vi "read-write user data.vi"(7 "Function":enum16{"Read", "Write"}(ring), 8 "error in (no error)":errorcluster, 10 "user data in":T1={"sectors"=[], "key names"=[], "values"=[]}, 11 "file name":string) -> (0 "error out":errorcluster, 2 "user data out":T1)   [LabVIEW 2015]
doc: "This VI saves (Write) and retrieves (Read) data from a configuration .ini file, regardless of the number of sectors and the keys in each sector."
uses:
  <vilib>/Utility/config.llb/NI_LVConfig.lvlib
  <vilib>/Utility/config.llb/Read Key (String).vi
  <vilib>/Utility/config.llb/Write Key (String).vi
  controls/user data.ctl
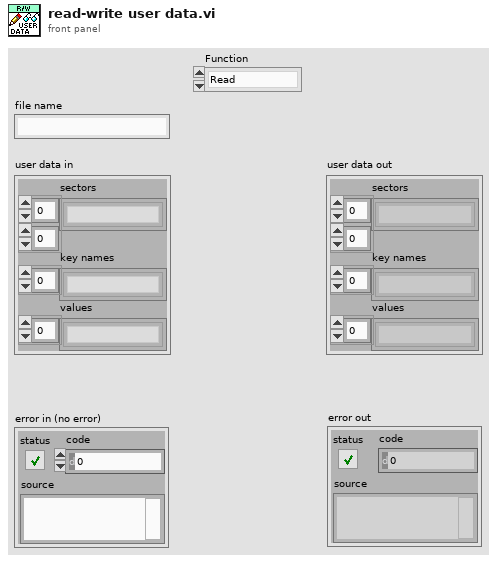
[diagram p1: front panel]
types:
  T1 = typedef "user data.ctl" = cluster{"sectors":string[][], "key names":string[], "values":string[]}
  T2 = typedef "NI_LVConfig.lvlib/Config Data RefNum.ctl" = refnum<k1>
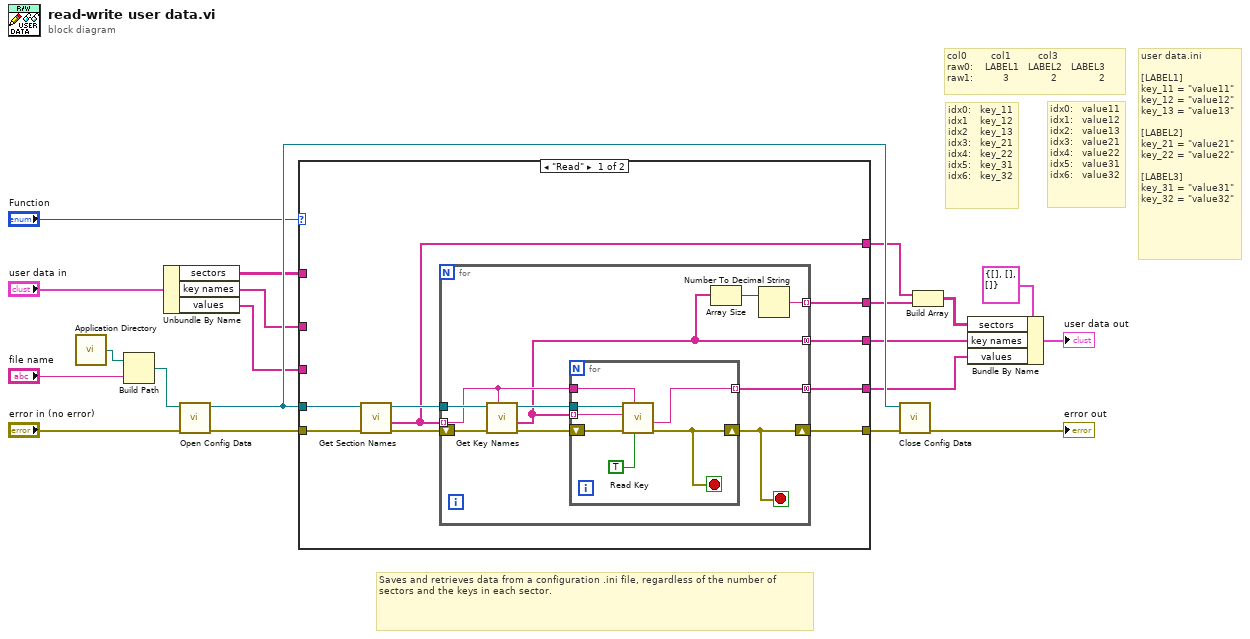
[diagram p0: block diagram]
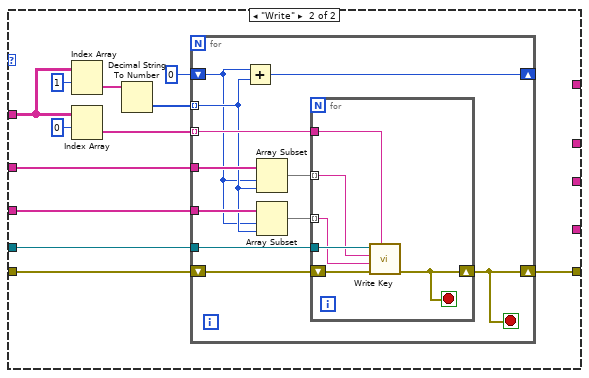
[diagram p2: hidden frame]
diagram:
  # "user data.ini\n\n[LABEL1]\nkey_11 = \"value11\"\nkey_12 = \"value12\"\nkey_13 = \"value13\"\n\n[LABEL2]\nkey_21 = \"value21\"\nkey_22 = \"value22\"\n\n[LABEL3]\nkey_31 = \"value31\"\nkey_32 = \"value32\""
  # "idx0:   value11\nidx1:   value12\nidx2:   value13\nidx3:   value21\nidx4:   value22\nidx5:   value31\nidx6:   value32"
  # "idx0:   key_11\nidx1    key_12\nidx2    key_13\nidx3:   key_21\nidx4:   key_22\nidx5:   key_31\nidx6:   key_32"
  # "col0        col1         col3   \nraw0:    LABEL1   LABEL2   LABEL3\nraw1:          3              2              2"
  # "Saves and retrieves data from a configuration .ini file, regardless of the number of sectors and the keys in each sector."
  n1 = call <vilib>:"Application Directory.vi"() -> ("Application Directory"=w16:path)
  n2 = Build Path(base path=w16, name or relative path="file name") -> (appended path=w18:path)
  n3 = Unbundle By Name("user data in") -> ("sectors"=w1:string[][], "key names"=w5:string[], "values"=w4:string[])
  n4 = call <vilib>:"Open Config Data.vi"("error in (no error)"="error in (no error)", "configuration file path"=w18) -> ("error out"=w20:errorcluster, "refnum"=w13:T2)  [unwired: 7 in, 1 out]
  n5 = case shown="\"Read\"" "Function" {
    tunnel: w20 -> [w27 w58]
    tunnel: [w26 w57] -> w15
    tunnel: w13 -> [w25 w55]
    tunnel: [w22 _] -> w9
    tunnel: [w24 _] -> w11
    tunnel: [w23 _] -> w10
    tunnel: w1 -> [_ w51]
    tunnel: w4 -> [_ w56]
    tunnel: w5 -> [_ w47]
    tunnel: [w21 _] -> w8
    frame "Read" {
      n6 = call <vilib>:"Get Section Names.vi"("error in (no error)"=w27, "refnum"=w25) -> ("error out"=w28:errorcluster, "section names"=w22:string[], "refnum out"=w29:T2)  [unwired: 7 in]
      n7 = for {
        tunnel: w29 -> [w39]
        tunnel: w22 -> [w33] mode=indexing
        shift-right: [w35] -> w26
        shift-left: w28 -> [w38]
        tunnel: [w32] -> w24 mode=concatenating
        tunnel: [w34] -> w23 mode=concatenating
        tunnel: [w30] -> w21 mode=indexing
        stop <- w35 stop-if-true
        n8 = call <vilib>:"Get Key Names.vi"("section"=w33, "error in (no error)"=w38, "refnum"=w39) -> ("error out"=w37:errorcluster, "key names"=w32:string[], "refnum out"=w36:T2)  [unwired: 5 in, 1 out]
        n9 = for {
          shift-right: [w41] -> w35
          shift-left: w37 -> [w46]
          tunnel: w32 -> [w42] mode=indexing
          tunnel: w36 -> [w45]
          tunnel: w33 -> [w44]
          tunnel: [w43] -> w34 mode=indexing
          stop <- w41 stop-if-true
          n10 = call-poly <vilib>:"Read Key.vi"("read raw string? (F)"=TRUE, "section"=w44, "error in (no error)"=w46, "key"=w42, "refnum"=w45) -> ("error out"=w41:errorcluster, "value"=w43:string)  [unwired: 3 in, 2 out]
        }
        n11 = Array Size(array=w32) -> (size(s)=w31:i32)
        n12 = Number To Decimal String(number=w31) -> (decimal integer string=w30:string)  [unwired: 1 in]
      }
    }
    frame "Write" {
      n13 = Index Array(array=w51, index (row)=1) -> (element=w50:string[])  [unwired: 1 in]
      n14 = Index Array(array=w51, index (row)=0) -> (element=w53:string[])  [unwired: 1 in]
      n15 = Decimal String To Number(string=w50) -> (number=w49:i32[])  [unwired: 2 in, 1 out]
      n16 = for {
        tunnel: w56 -> [w62]
        tunnel: w47 -> [w65]
        tunnel: w55 -> [w68]
        tunnel: w53 -> [w67] mode=indexing
        shift-right: [w66] -> w57
        shift-left: w58 -> [w69]
        tunnel: w49 -> [w60] mode=indexing
        shift-right: [w63] -> _
        shift-left: 0 ("sector") -> [w59]
        stop <- w66 stop-if-true
        n17 = Add(x=w59, y=w60) -> (x+y=w63:i32)
        n18 = Array Subset(array=w65, index=w59, length=w60) -> (w64:string[])
        n19 = Array Subset(array=w62, index=w59, length=w60) -> (w61:string[])
        n20 = for {
          tunnel: w68 -> [w75]
          shift-right: [w70] -> w66
          shift-left: w69 -> [w74]
          tunnel: w67 -> [w73]
          tunnel: w64 -> [w72] mode=indexing
          tunnel: w61 -> [w71] mode=indexing
          stop <- w70 stop-if-true
          n21 = call-poly <vilib>:"Write Key.vi"("section"=w73, "error in (no error)"=w74, "value"=w71, "key"=w72, "refnum"=w75) -> ("error out"=w70:errorcluster)  [unwired: 4 in, 2 out]
        }
      }
    }
  }
  n22 = call <vilib>:"Close Config Data.vi"("error in (no error)"=w15, "refnum"=w13) -> ("error out"=→"error out":errorcluster)  [unwired: 8 in, 1 out]
  n23 = Build Array(w9, w8) -> (w7:string[][])
  n24 = Bundle By Name(cluster=T1 {"sectors"=[], "key names"=[], "values"=[]} ("user data out"), "sectors"=w7, "key names"=w11, "values"=w10) -> (→"user data out":T1)
